vi "VAT_valve_initialise.vi"(0 "VAT Valve COM port":refnum<visa-resource-name>, 11 "error in (no error)":errorcluster) -> (4 "VAT Valve COM port out":refnum<visa-resource-name>, 6 "Temperature":dbl, 8 "Status":dbl, 10 "Version":dbl, 12 "Software Version":dbl, 13 "Valve Type":string, 14 "Position":dbl, 15 "error out":errorcluster)   [LabVIEW 2019]
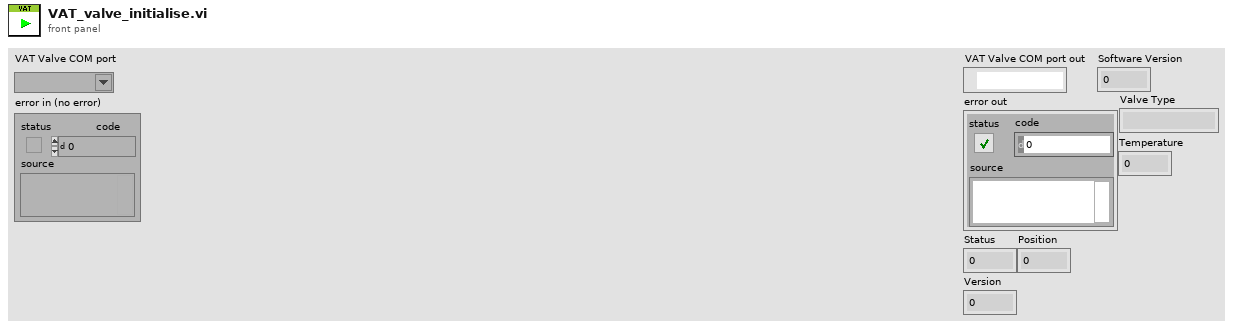
[diagram p1: front panel]
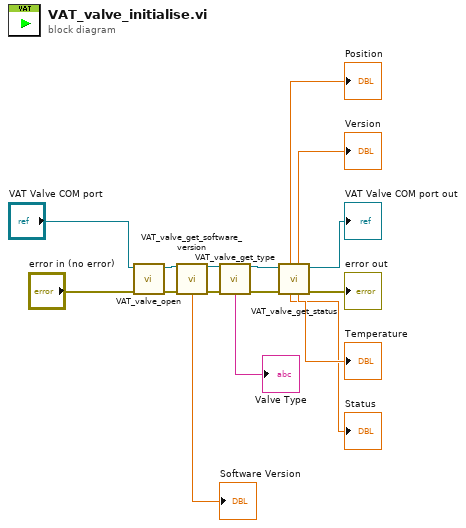
[diagram p0: block diagram]
diagram:
  n1 = call "VAT_valve_open.vi"("error in (no error)"="error in (no error)", "VAT Valve COM port"="VAT Valve COM port") -> ("error out"=w15:errorcluster, "VISA resource name out"=w16:refnum<visa-resource-name>)  [unwired: 8 in]
  n2 = call "VAT_valve_get_software_version.vi"("VAT Valve COM port"=w16, "error in (no error)"=w15) -> ("VAT Valve COM port out"=w14:refnum<visa-resource-name>, "Software Version"=→"Software Version":dbl, "error out"=w13:errorcluster)  [unwired: 11 in]
  n3 = call "VAT_valve_get_type.vi"("VAT Valve COM port"=w14, "error in (no error)"=w13) -> ("VAT Valve COM port out"=w12:refnum<visa-resource-name>, "Valve Type"=→"Valve Type":string, "error out"=w11:errorcluster)  [unwired: 11 in]
  n4 = call "VAT_valve_get_status.vi"("error in (no error)"=w11, "VAT Valve COM port"=w12) -> ("error out"=→"error out":errorcluster, "VAT Valve COM port out"=→"VAT Valve COM port out":refnum<visa-resource-name>, "Temperature"=→"Temperature":dbl, "Version"=→"Version":dbl, "Status"=→"Status":dbl, "Position"=→"Position":dbl)  [unwired: 4 in]
